vi "Init.vi"(8 "error in (no error)":errorcluster, 10 "ID":string, 11 "Channel in":refnum<class "Channel.lvclass">) -> (0 "error out":errorcluster, 3 "Channel out":refnum<class "Channel.lvclass">)   [LabVIEW 2019, in "Channel.lvclass"]
uses:
  Channel.lvclass
  EQ.ctl
  Libraries/Audio Processing/Value Cluster.ctl
  Libraries/Audio Processing/Value Properties.ctl
  Channel.lvclass/Channel.ctl
  Effect/Effect.lvclass
  Libraries/Messaging/Messaging.lvlib
  Libraries/Audio Processing/Audio Processing.lvlib
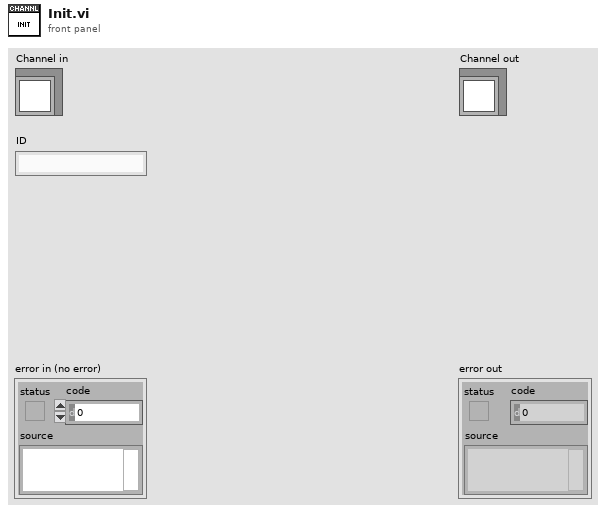
[diagram p1: front panel]
types:
  T1 = typedef "Audio Processing.lvlib/Value Cluster.ctl" = cluster{"Value":dbl, "Limits":T2}
  T2 = typedef "Audio Processing.lvlib/Value Properties.ctl" = cluster{"Lower":dbl, "Upper":dbl}
  T3 = typedef "Channel.lvclass/EQ.ctl" = cluster{"Level":T1, "Kill":bool}
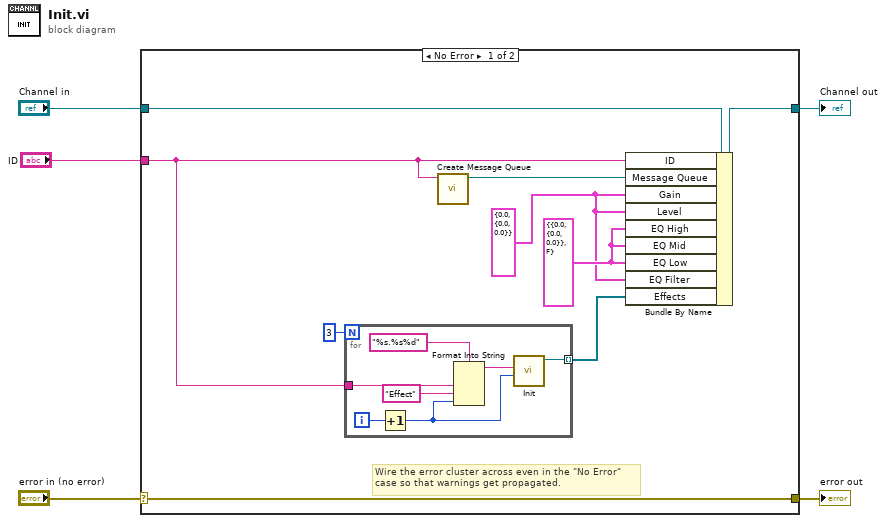
[diagram p0: block diagram]
diagram:
  n1 = case shown="No Error" "error in (no error)" {
    selector: "error in (no error)" -> [w14 w23]
    tunnel: [w14 w23] -> w4
    tunnel: [w13 w22] -> w2
    tunnel: "Channel in" -> [w12 w22]
    tunnel: "ID" -> [w9 _]
    frame No Error {
      w6 = T1 {"Value"=0.0, "Limits"={"Lower"=0.0, "Upper"=0.0}} ("Level")
      w7 = T3 {"Level"={"Value"=0.0, "Limits"={"Lower"=0.0, "Upper"=0.0}}, "Kill"=FALSE} ("EQ High")
      # "Wire the error cluster across even in the \"No Error\"\ncase so that warnings get propagated."
      n2 = for {
        N: 3 -> [_]
        tunnel: w9 -> [w21]
        tunnel: [w16] -> w10 mode=indexing
        i -> [w19]
        n3 = Increment(x=w19) -> (x+1=w15:i32)
        n4 = Format Into String(format string="%s.%s%d", w21, "Effect" ("input 2"), w15) -> (resulting string=w17:string)  [unwired: 2 in, 1 out]
        n5 = call "Init.vi"("Type"=w15, "ID"=w17) -> ("Effect out"=w16:refnum<class "Effect.lvclass">)  [unwired: 8 in, 1 out]
      }
      n6 = call "Create Message Queue.vi"("Queue Name"=w9) -> ("queue out"=w8:refnum<queue>)  [unwired: 9 in, 1 out]
      n7 = Bundle By Name(cluster=w12, "ID"=w9, "Message Queue"=w8, "Gain"=w6, "Level"=w6, "EQ High"=w7, "EQ Mid"=w7, "EQ Low"=w7, "EQ Filter"=w6, "Effects"=w10) -> (w13:refnum<class "Channel.lvclass">)
    }
    frame Error {
    }
  }
  "error out" <- w4
  "Channel out" <- w2
